vi "Determine Warnings-Edit.vi"() -> ()   [LabVIEW 2014]
panel:
  out "Warning?":bool
  out "Warning Text":string
  in  "Min Temp":dbl
  in  "Max Temp":dbl
  in  "Current Temp":dbl
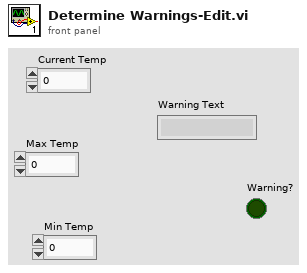
[diagram p1: front panel]
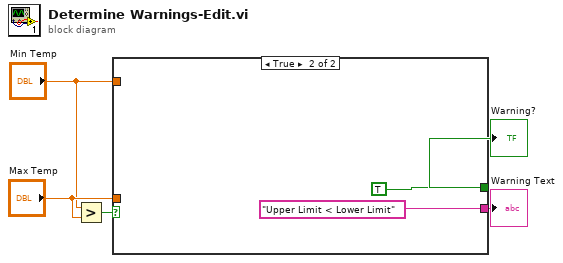
[diagram p0: block diagram]
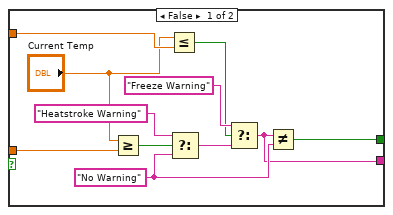
[diagram p2: hidden frame]
diagram:
  n1 = Greater?(x="Min Temp", y="Max Temp") -> (0:w3:bool)
  n2 = case shown="True" w3 {
    tunnel: "Min Temp" -> [w16 _]
    tunnel: "Max Temp" -> [w14 _]
    tunnel: [w7 TRUE] -> w2
    tunnel: [w6 "Upper Limit < Lower Limit"] -> w1
    frame False {
      w13 = "No Warning"
      n3 = Greater Or Equal?(x="Current Temp", y=w14) -> (x >= y?=w9:bool)
      n4 = Less Or Equal?(x="Current Temp", y=w16) -> (x <= y?=w8:bool)
      n5 = Select(t="Heatstroke Warning", s=w9, f=w13) -> (s? t:f=w12:string)
      n6 = Select(t="Freeze Warning", s=w8, f=w12) -> (s? t:f=w6:string)
      n7 = Not Equal?(x=w6, y=w13) -> (x != y?=w7:bool)
    }
    frame True {
    }
  }
  "Warning Text" <- w1
  "Warning?" <- w2
